vi "Gen Trigger Pulse.vi"(0 "Threshold In":bool) -> (3 "Threshold Out":bool)   [LabVIEW 2017]
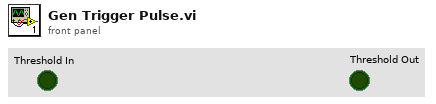
[diagram p1: front panel]
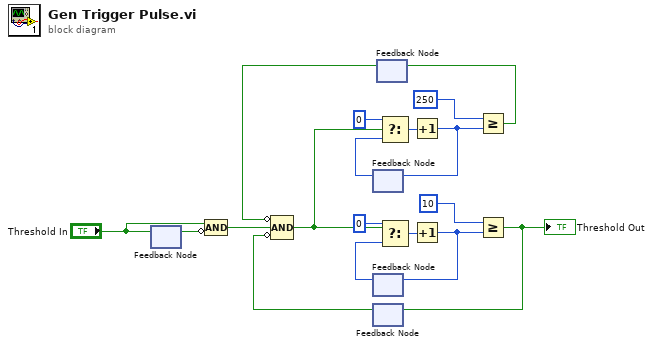
[diagram p0: block diagram]
diagram:
  n1 = feedback-in #1("Threshold In") -> ()
  n2 = feedback #1() -> (w18:bool)  [unwired: 1 in]
  n3 = Compound Arithmetic op=AND("Threshold In", invert w18) -> (w16:bool)
  n4 = feedback #2() -> (w6:i64)  [unwired: 1 in]
  n5 = feedback #3() -> (w13:i64)  [unwired: 1 in]
  n6 = feedback #4() -> (w10:bool)  [unwired: 1 in]
  n7 = feedback #5() -> (w1:bool)  [unwired: 1 in]
  n8 = Compound Arithmetic op=AND(invert w1, w16, invert w10) -> (w3:bool)
  n9 = Select(t=i64 0, s=w3, f=w6) -> (s? t:f=w5:i64)
  n10 = Select(t=i64 0, s=w3, f=w13) -> (s? t:f=w14:i64)
  n11 = Increment(x=w5) -> (x+1=w7:i64)
  n12 = feedback-in #2(w7) -> ()
  n13 = Increment(x=w14) -> (x+1=w12:i64)
  n14 = feedback-in #3(w12) -> ()
  n15 = Greater Or Equal?(x=i64 250, y=w7) -> (x >= y?=w2:bool)
  n16 = feedback-in #5(w2) -> ()
  n17 = Greater Or Equal?(x=i64 10, y=w12) -> (x >= y?=w9:bool)
  "Threshold Out" <- w9
  n18 = feedback-in #4(w9) -> ()
